vi "Direct.vi"(7 "Actor in":refnum<class "Actor.lvclass">) -> (0 "Error out":errorcluster, 5 "Actor out":refnum<class "Actor.lvclass">)   [LabVIEW 2025, in "_Template.lvlib" / "Templates.lvlib" / "TEMPLATE Msg.lvlib"]
uses:
  TEMPLATE Msg.lvlib
  jettl/jettl/Actor/Actor/Actor.lvclass
  TEMPLATE Msg/TEMPLATE Msg.lvclass
  jettl/jettl/Actor/Actor.lvlib
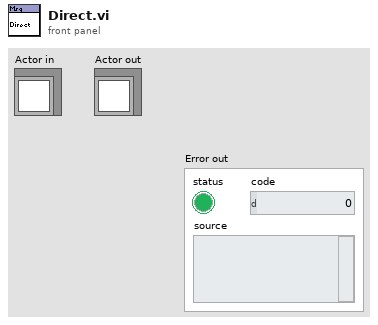
[diagram p1: front panel]
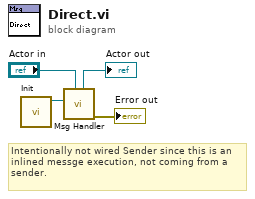
[diagram p0: block diagram]
diagram:
  # "Intentionally not wired Sender since this is an inlined messge execution, not coming from a sender."
  n1 = call "Init.vi"() -> ("TEMPLATE Msg out"=w2:refnum<class "TEMPLATE Msg.lvclass">)  [unwired: 11 in]
  n2 = call "Msg Handler.vi"("Actor in"="Actor in", "Msg"=w2) -> ("Error out"=→"Error out":errorcluster, "Actor out"=→"Actor out":refnum<class "Actor.lvclass">)  [unwired: 8 in]
